vi "GetStructureTunnels.vi"(5 "Structure in":refnum<class "Structure.lvclass">, 6 "error in":errorcluster, 9 "VI Interpreter in":refnum<class "VI Interpreter.lvclass">) -> (0 "error out":errorcluster, 3 "VI Interpreter out":refnum<class "VI Interpreter.lvclass">, 4 "Structure out":refnum<class "Structure.lvclass">)   [LabVIEW 2014, in "VI Interpreter.lvclass"]
uses:
  VI Interpreter.lvclass
  Structure/Structure.lvclass
  Structure/Structure.lvclass/Structure.ctl
  Tunnel/Tunnel.lvclass
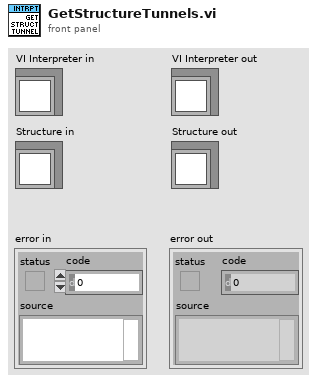
[diagram p1: front panel]
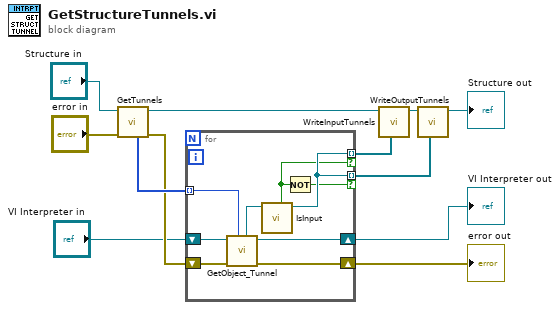
[diagram p0: block diagram]
diagram:
  n1 = call-dynamic "GetTunnels.vi"("error in"="error in", "Structure in"="Structure in") -> ("error out"=w11:errorcluster, "Structure out"=w5:refnum<class "Structure.lvclass">, "Tunnels"=w12:i32[])  [unwired: 5 in]
  n2 = for {
    shift-right: [w17] -> w10
    shift-left: "VI Interpreter in" -> [w21]
    tunnel: w12 -> [w20] mode=indexing
    shift-right: [w19] -> w9
    shift-left: w11 -> [w18]
    tunnel: [w15] -> w2 mode=indexing if=w13
    tunnel: [w15] -> w4 mode=indexing if=w14
    n3 = call "GetObject_Tunnel.vi"("UID"=w20, "error in"=w18, "VI Interpreter in"=w21) -> ("error out"=w19:errorcluster, "VI Interpreter out"=w17:refnum<class "VI Interpreter.lvclass">, "Tunnel"=w16:refnum<class "Tunnel.lvclass">)  [unwired: 3 in, 1 out]
    n4 = call "IsInput.vi"("Tunnel in"=w16) -> ("Tunnel out"=w15:refnum<class "Tunnel.lvclass">, "Input"=w14:bool)  [unwired: 6 in, 1 out]
    n5 = Not(x=w14) -> (.not. x?=w13:bool)
  }
  "error out" <- w9
  "VI Interpreter out" <- w10
  n6 = call "WriteInputTunnels.vi"("inputs"=w4, "Structure in"=w5) -> ("Structure out"=w3:refnum<class "Structure.lvclass">)  [unwired: 7 in]
  n7 = call-dynamic "WriteOutputTunnels.vi"("outputs"=w2, "Structure in"=w3) -> ("Structure out"=→"Structure out":refnum<class "Structure.lvclass">)  [unwired: 7 in]
